vi "Default User Interface.vi"(8 "error in (no error)":errorcluster, 11 "User Interface in":refnum<class "User Interface.lvclass">) -> (0 "error out":errorcluster, 3 "User Interface out":refnum<class "User Interface.lvclass">)   [LabVIEW 2020, in "DSF Core.lvlib" / "User Interface.lvclass"]
uses:
  User Interface.lvclass
  Configuration/Configuration.lvclass
panel:
  # "No settings required."
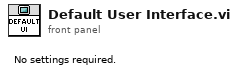
[diagram p1: front panel]
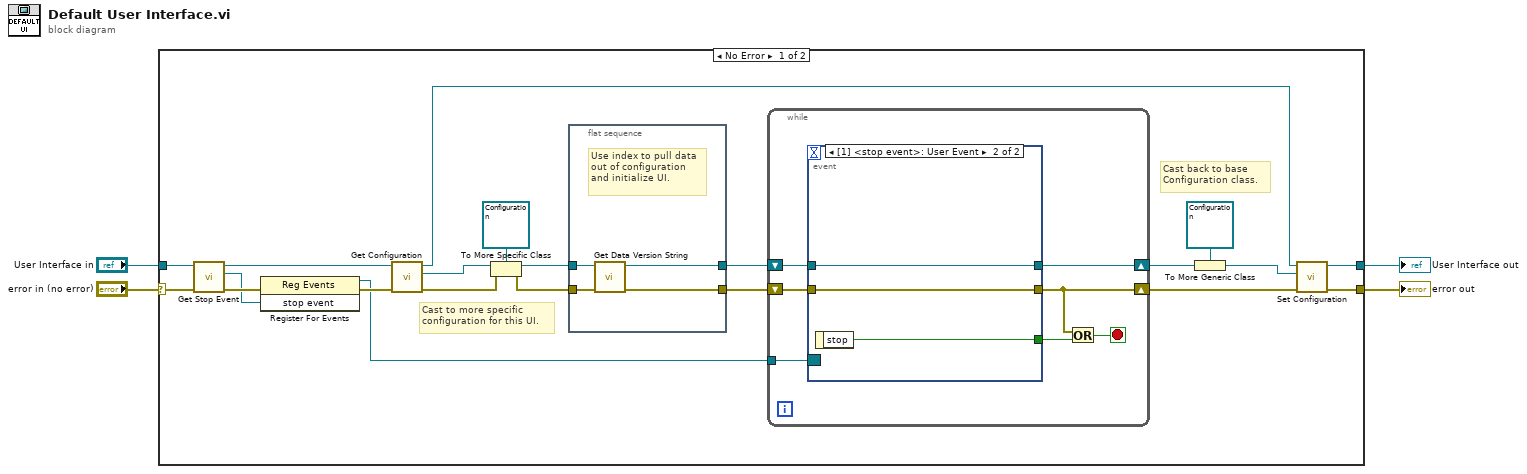
[diagram p0: block diagram]
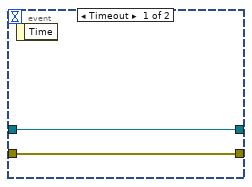
[diagram p2: hidden frame]
diagram:
  n1 = case shown="No Error" "error in (no error)" {
    selector: "error in (no error)" -> [w21 w43]
    tunnel: [w7 w43] -> w4
    tunnel: "User Interface in" -> [w20 w42]
    tunnel: [w6 w42] -> w1
    frame No Error {
      # "Cast back to base Configuration class."
      # "Cast to more specific configuration for this UI."
      n2 = call "Get Stop Event.vi"("error in (no error)"=w21, "User Interface in"=w20) -> ("error out"=w19:errorcluster, "stop event"=w18:refnum<user-event>, "User Interface out"=w17:refnum<class "User Interface.lvclass">)  [unwired: 7 in]
      n3 = register-events(error in=w19, w18) -> (reference out=w15:refnum<event-registration>, error out=w16:errorcluster)  [unwired: 1 in]
      n4 = call "Get Configuration.vi"("error in (no error)"=w16, "User Interface in"=w17) -> ("error out"=w14:errorcluster, "configuration"=w12:refnum<class "Configuration.lvclass">, "User Interface out"=w5:refnum<class "User Interface.lvclass">)  [unwired: 7 in]
      n5 = To More Specific Class(target class=refnum<class "Configuration.lvclass"> refnum ("Configuration out"), reference=w12, error in=w14) -> (specific class reference=w25:refnum<class "Configuration.lvclass">, error out=w22:errorcluster)
      n6 = flat-sequence {
        tunnel: [w27] -> w23
        tunnel: w22 -> [w29]
        tunnel: w25 -> [w28]
        tunnel: [w26] -> w24
        frame #0 {
          # "Use index to pull data out of configuration and initialize UI."
          n7 = call "Get Data Version String.vi"("error in (no error)"=w29, "Configuration in"=w28) -> ("error out"=w27:errorcluster, "Configuration out"=w26:refnum<class "Configuration.lvclass">)  [unwired: 7 in, 1 out]
        }
      }
      n8 = while {
        tunnel: w15 -> [w36]
        shift-right: [w34] -> w9
        shift-left: w23 -> [w35]
        shift-right: [w30] -> w11
        shift-left: w24 -> [w31]
        stop <- w33 stop-if-true
        n9 = event shown="[1] <stop event>: User Event" {
          selector: w36 -> [_ _]
          dyn-events: _ -> [_ _]
          timeout: _ -> [_ _]
          tunnel: [_ w39] -> w32
          tunnel: w35 -> [w38 w41]
          tunnel: [w38 w41] -> w34
          tunnel: w31 -> [w37 w40]
          tunnel: [w37 w40] -> w30
          event Timeout {
            n10 = event-data() -> ()  [unwired: 1 in, 1 out]
          }
          event User Event {
            n11 = event-data() -> ("stop"=w39:bool)  [unwired: 1 in]
          }
        }
        n12 = Or(x=w34, y=w32) -> (x .or. y?=w33:bool)
      }
      n13 = To More Generic Class(target class=refnum<class "Configuration.lvclass"> refnum ("Configuration out"), reference=w11) -> (generic class reference=w8:refnum<class "Configuration.lvclass">)
      n14 = call "Set Configuration.vi"("error in (no error)"=w9, "configuration"=w8, "User Interface in"=w5) -> ("error out"=w7:errorcluster, "User Interface out"=w6:refnum<class "User Interface.lvclass">)  [unwired: 7 in]
    }
    frame Error {
    }
  }
  "error out" <- w4
  "User Interface out" <- w1
